vi "Calculate Leak Rate.vi"(8 "error in (no error)":errorcluster, 9 "Count":i32, 10 "Averaged Values":dbl[](array[numeric]), 11 "Buffer":dbl[][](array[numeric])) -> (0 "error out":errorcluster, 3 "Values":dbl[](array[numeric]))   [LabVIEW 2015]
doc: "This VI implements a moving average filter for this particular channel"
uses:
  <vilib>/Analysis/NI_AALPro.lvlib
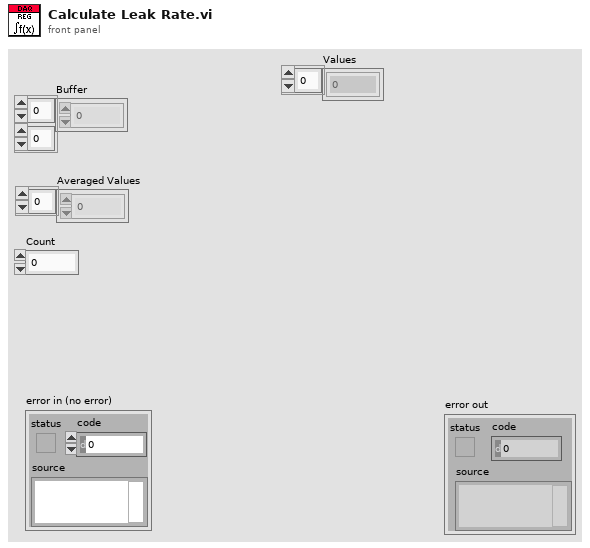
[diagram p1: front panel]
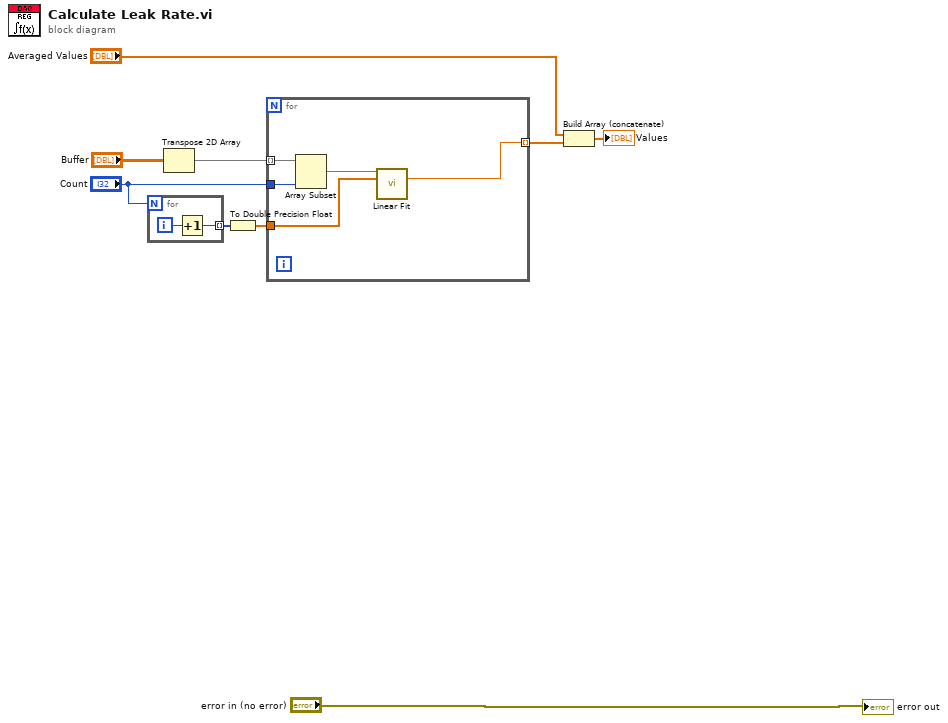
[diagram p0: block diagram]
diagram:
  n1 = for {
    N: "Count" -> [_]
    tunnel: [w10] -> w6 mode=indexing
    i -> [w11]
    n2 = Increment(x=w11) -> (x+1=w10:i32)
  }
  n3 = Transpose 2D Array(2D array="Buffer") -> (transposed array=w2:dbl[][])
  n4 = To Double Precision Float(number=w6) -> (double precision float=w5:dbl[])
  n5 = for {
    tunnel: w2 -> [w16] mode=indexing
    tunnel: "Count" -> [w13]
    tunnel: w5 -> [w14]
    tunnel: [w12] -> w1 mode=indexing
    n6 = Array Subset(array=w16, length=w13) -> (w15:dbl[])  [unwired: 1 in]
    n7 = call <vilib>:"Linear Fit.vi"("Y"=w15, "X"=w14) -> ("slope"=w12:dbl)  [unwired: 9 in, 4 out]
  }
  n8 = Build Array (concatenate)("Averaged Values", w1) -> (→"Values":dbl[])
  "error out" <- "error in (no error)"
